vi "CS-4 Set Switch Heater.vi"(4 "error in (no error)":errorcluster, 6 "switch heater":bool, 7 "VISA session":refnum<visa-resource-name>) -> (0 "error out":errorcluster, 3 "dup VISA session":refnum<visa-resource-name>)   [LabVIEW 2016]
doc: "CS-4 Set Switch Heater.vi will turn the switch heater on or off per the boolean input."
panel:
  # "On"
  # "Off"
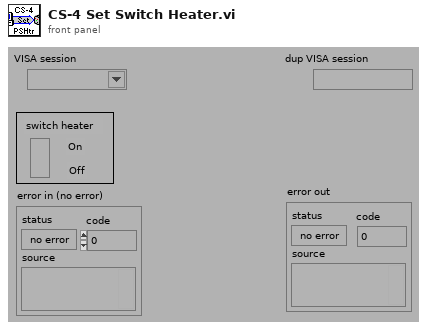
[diagram p1: front panel]
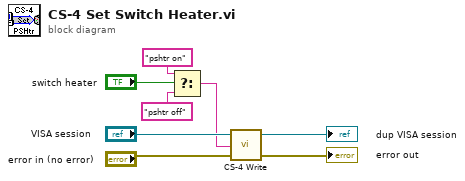
[diagram p0: block diagram]
diagram:
  n1 = Select(t="pshtr on", s="switch heater", f="pshtr off") -> (s? t:f=w3:string)
  n2 = call "CS-4 Write.vi"("error in (no error)"="error in (no error)", "write buffer (\"\")"=w3, "VISA session"="VISA session") -> ("error out"=→"error out":errorcluster, "dup VISA session"=→"dup VISA session":refnum<visa-resource-name>)  [unwired: 1 out]
